vi "Open.vi"(8 "error in (no error)":errorcluster, 9 "Mode":T1, 10 "Data Source":string, 11 "Sqlite Database Manager in":refnum<class "Sqlite Database Manager.lvclass">) -> (0 "error out":errorcluster, 3 "Sqlite Database Manager out":refnum<class "Sqlite Database Manager.lvclass">)   [LabVIEW 2019, in "HierDAL Library.lvlib" / "Database.lvlib" / "Sqlite Database Manager.lvclass"]
doc: "Opens a database on disk and initialises it.\n \n<b>Path</b> - Paths to the database on disk.\n<b>Mode</b> - The mode of operation (e.g., Create, Replace, Open, ReadOnly).\n <b>Create</b> - Creates a new database. If the database file already exists, it will be overwritten.\n <b>Replace</b> - Replaces the existing database with a new one.\n <b>Open</b> - Opens an existing database without modifying it.\n <b>Read Only</b> - Opens the database in read-only mode."
uses:
  Sqlite Database Manager.lvclass
  Database Manager Class/Controls/Mode.ctl
  System.Data.SQLite
  Sqlite Database Manager.lvclass/Sqlite Database Manager.ctl
  Database Manager Class/Database Manager.lvclass
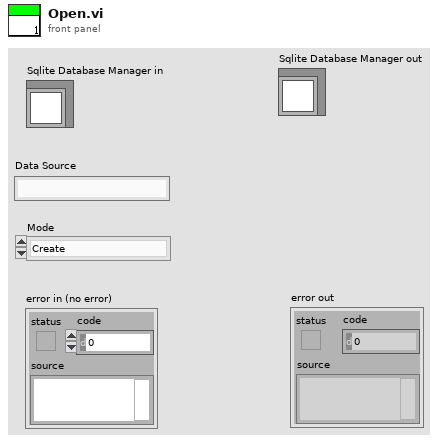
[diagram p1: front panel]
types:
  T1 = typedef "HierDAL Library.lvlib/Database.lvlib/Database Manager.lvclass/Mode.ctl" = enum16{"Create", "Replace", "Open", "Read Only"}
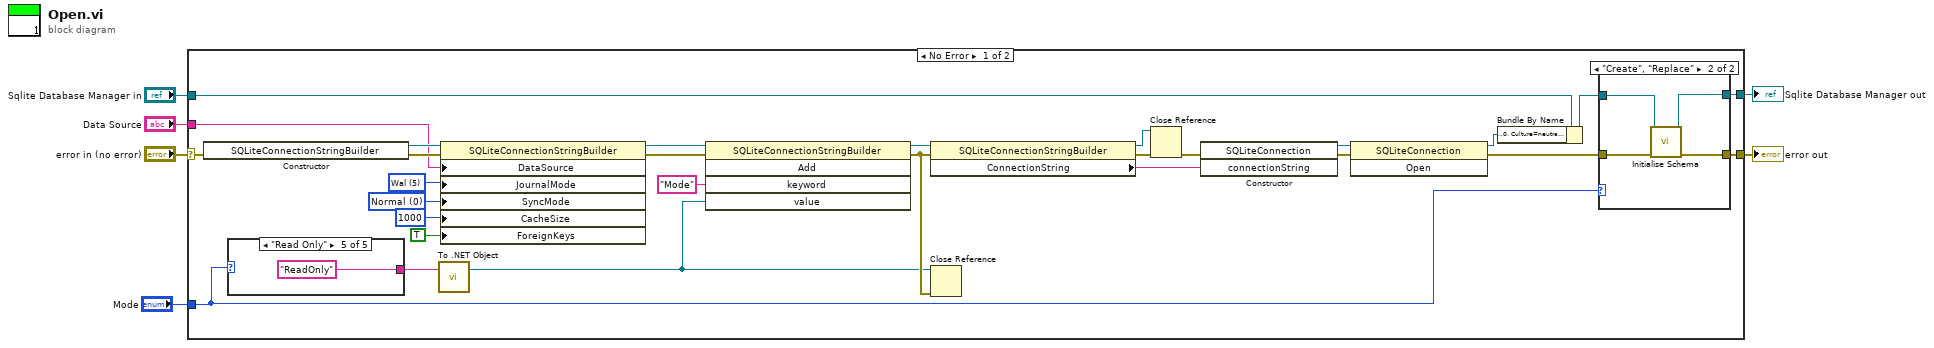
[diagram p0: block diagram]
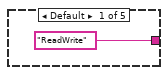
[diagram p3: hidden frame]
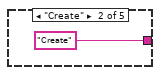
[diagram p4: hidden frame]
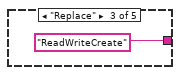
[diagram p5: hidden frame]
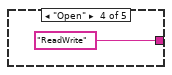
[diagram p6: hidden frame]
diagram:
  n1 = case shown="No Error" "error in (no error)" {
    selector: "error in (no error)" -> [w19 w46]
    tunnel: "Data Source" -> [w24 _]
    tunnel: [w13 w46] -> w5
    tunnel: "Sqlite Database Manager in" -> [w18 w47]
    tunnel: [w15 w47] -> w2
    tunnel: "Mode" -> [w14 _]
    frame No Error {
      w20 = 5 items=["Delete"=0, "Persist"=1, "Off"=2, "Truncate"=3, "Memory"=4, "Wal"=5, "Default"=-1] ("JournalMode")
      w21 = 0 items=["Normal", "Full", "Off"] ("SyncMode")
      n2 = constructor class="SQLiteConnectionStringBuilder"(error in=w19) -> (reference out=w33:refnum<k24>, error out=w34:errorcluster)  [unwired: 2 in, 1 out]
      n3 = case shown="\"Read Only\"" w14 {
        tunnel: ["ReadWrite" "Create" "ReadWriteCreate" "ReadWrite" "ReadOnly"] -> w17
        frame Default {
        }
        frame "Create" {
        }
        frame "Replace" {
        }
        frame "Open" {
        }
        frame "Read Only" {
        }
      }
      n4 = call <vilib>:"To .NET Object.vi"("anything"=w17) -> (".NET object"=w11:refnum<k24>)  [unwired: 1 in, 1 out]
      n5 = property class="SQLiteConnectionStringBuilder"(reference=w33, error in=w34, "DataSource"=w24, "JournalMode"=w20, "SyncMode"=w21, "CacheSize"=1000, "ForeignKeys"=TRUE) -> (reference out=w31:refnum<k24>, error out=w32:errorcluster)
      n6 = invoke class="SQLiteConnectionStringBuilder" method="Add"(reference=w31, error in=w32, "keyword"="Mode", "value"=w11) -> (reference out=w30:refnum<k24>, error out=w12:errorcluster)  [unwired: 1 in, 3 out]
      n7 = property class="SQLiteConnectionStringBuilder"(reference=w30, error in=w12) -> (reference out=w28:refnum<k24>, error out=w29:errorcluster, "ConnectionString"=w26:string)
      n8 = Close Reference(reference=w11, error in (no error)=w12) -> ()  [unwired: 1 out]
      n9 = Close Reference(reference=w28, error in (no error)=w29) -> (error out=w27:errorcluster)
      n10 = constructor class="SQLiteConnection"(error in=w27, "connectionString"=w26) -> (reference out=w9:refnum<k24>, error out=w10:errorcluster)  [unwired: 2 in, 2 out]
      n11 = invoke class="SQLiteConnection" method="Open"(reference=w9, error in=w10) -> (reference out=w7:refnum<k24>, error out=w8:errorcluster)  [unwired: 1 in, 1 out]
      n12 = Bundle By Name(cluster=w18, "Connection"=w7) -> (w16:refnum<class "Sqlite Database Manager.lvclass">)
      n13 = case shown="\"Create\", \"Replace\"" w14 {
        tunnel: w8 -> [w35 w40]
        tunnel: w16 -> [w36 w39]
        tunnel: [w36 w38] -> w15
        tunnel: [w35 w37] -> w13
        frame Default {
        }
        frame "Create", "Replace" {
          n14 = call "Initialise Schema.vi"("error in (no error)"=w40, "Sqlite Database Manager in"=w39) -> ("error out"=w37:errorcluster, "Sqlite Database Manager out"=w38:refnum<class "Sqlite Database Manager.lvclass">)  [unwired: 8 in]
        }
      }
    }
    frame Error {
    }
  }
  "error out" <- w5
  "Sqlite Database Manager out" <- w2
